vi "Launch Step Configuration.vi"(8 "error in (no error)":errorcluster, 10 "Step Name":string, 11 "Controller in":refnum<class "Controller.lvclass">) -> (0 "error out":errorcluster, 3 "Controller out":refnum<class "Controller.lvclass">)   [LabVIEW 2017, in "Controller Actor.lvlib" / "Controller.lvclass"]
uses:
  Controller.lvclass
  C:/Program Files (x86)/National Instruments/LabVIEW 2017/vi.lib/ActorFramework/Actor/Actor.lvclass
  Measurement Actor/Measurement.lvclass/Measurement.ctl
  Measurement Actor/Configuration/Step Configuration.lvclass/Step Configuration.ctl
  Controller.lvclass/Controller.ctl
  Measurement Actor/Configuration/Step Configuration.lvclass
  Measurement Actor/Measurement.lvclass
  <vilib>/ActorFramework/Actor/Actor.lvclass
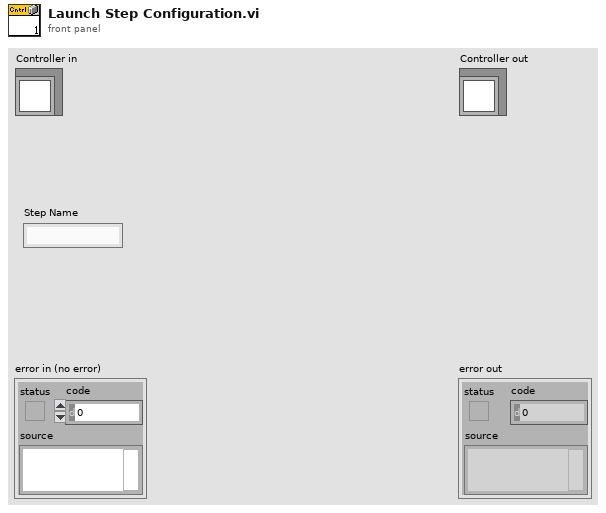
[diagram p1: front panel]
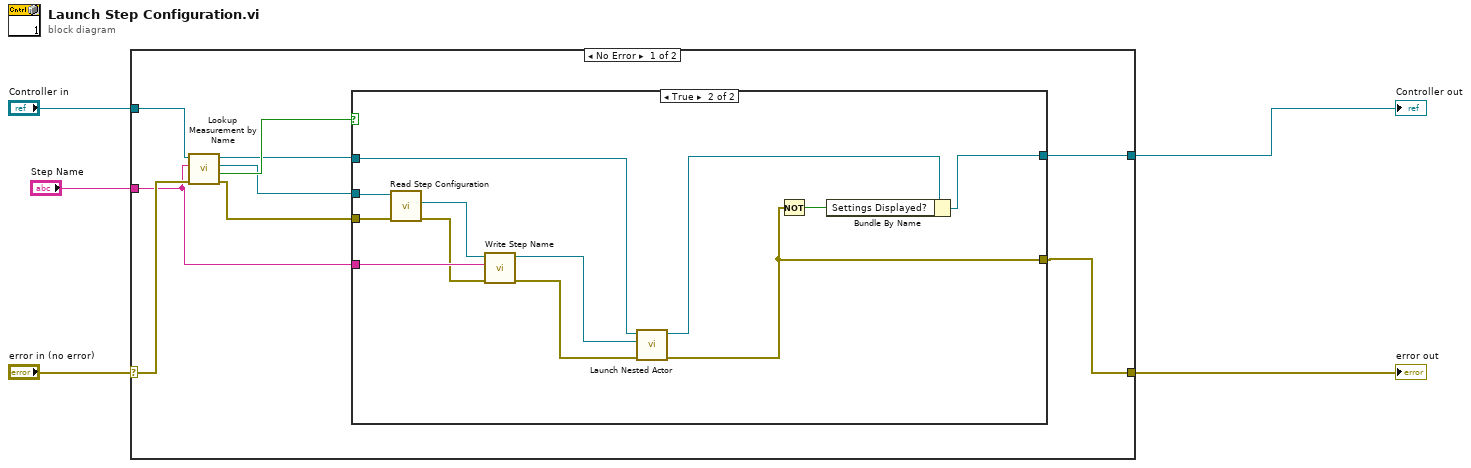
[diagram p0: block diagram]
diagram:
  n1 = case shown="No Error" "error in (no error)" {
    selector: "error in (no error)" -> [w13 w30]
    tunnel: [w12 w30] -> w4
    tunnel: [w8 w29] -> w2
    tunnel: "Controller in" -> [w9 w29]
    tunnel: "Step Name" -> [w11 _]
    frame No Error {
      n2 = call "Lookup Measurement by Name.vi"("error in (no error)"=w13, "Measurement Name"=w11, "Controller in"=w9) -> ("error out"=w14:errorcluster, "found"=w10:bool, "Measurement.lvclass"=w7:refnum<class "Measurement.lvclass">, "Controller out"=w6:refnum<class "Controller.lvclass">)  [unwired: 5 in]
      n3 = case shown="True" w10 {
        tunnel: w7 -> [_ w28]
        tunnel: w14 -> [w15 w27]
        tunnel: [w15 w21] -> w12
        tunnel: w11 -> [_ w26]
        tunnel: w6 -> [w16 w19]
        tunnel: [w16 w18] -> w8
        frame False {
        }
        frame True {
          n4 = call "Read Step Configuration.vi"("error in (no error)"=w27, "Measurement in"=w28) -> ("error out"=w24:errorcluster, "Measurement Actor.lvlib:Step Configuration.lvclass"=w25:refnum<class "Step Configuration.lvclass">)  [unwired: 7 in, 1 out]
          n5 = call "Write Step Name.vi"("error in (no error)"=w24, "Step Name"=w26, "Step Configuration in"=w25) -> ("error out"=w23:errorcluster, "Step Configuration out"=w20:refnum<class "Step Configuration.lvclass">)  [unwired: 7 in]
          n6 = call <vilib>:"Launch Nested Actor.vi"("error in (no error)"=w23, "Nested Actor"=w20, "Caller Actor in"=w19) -> ("error out"=w21:errorcluster, "Caller Actor out"=w17:refnum<class "Controller.lvclass">)  [unwired: 6 in, 1 out]
          n7 = Not(x=w21) -> (.not. x?=w22:bool)
          n8 = Bundle By Name(cluster=w17, "Settings Displayed?"=w22) -> (w18:refnum<class "Controller.lvclass">)
        }
      }
    }
    frame Error {
    }
  }
  "error out" <- w4
  "Controller out" <- w2
